vi "Set PORT levels.vi"(8 "error in (no error)":errorcluster, 9 "v (0.000000)":dbl, 10 "i (0)":T1, 11 "VISA resource name":refnum<visa-resource-name>) -> (0 "error out":errorcluster, 3 "VISA resource name out":refnum<visa-resource-name>)   [LabVIEW 2015, in "SR400.lvlib"]
doc: "PL i { ,v }\nThe PL command sets and reads thePORT1 and\nPORT2 output levels. i=1 or 2 to select PORT1 or\nPORT 2 and is required. If v is included, the\noutput level is set to v Volts where -10.000 <= v\n<= 10.000. The resolution is 0.005 V (5 mV). If v\nis absent, the output level is returned. If the Port\noutput mode is SCAN, the PL command sets and\nreads the starting value of the level. Changing the\nlevel during a scan will cause the level to be set to\nthe new value on the next count period. Note that\nthe scan is not reset. Reading the level during a\nscan always returns the starting value, not the\ncurrent value."
uses:
  SR400.lvlib
  Typedefs/PORT Output.ctl
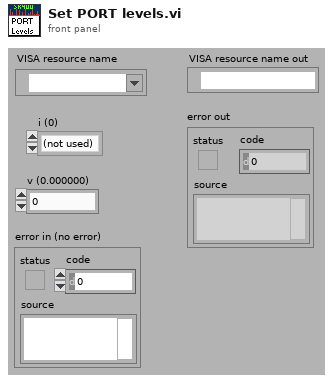
[diagram p1: front panel]
types:
  T1 = typedef "SR400.lvlib/PORT Output.ctl" = enum16{"(not used)", "PORT 1", "PORT 2"}
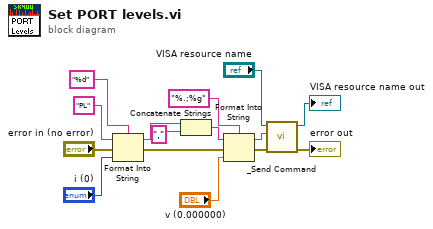
[diagram p0: block diagram]
diagram:
  n1 = Format Into String(format string="%d", initial string="PL" ("command"), error in="error in (no error)", "i (0)") -> (resulting string=w12:string, error out=w13:errorcluster)
  n2 = Concatenate Strings(w12, "," ("command")) -> (w7:string)
  n3 = Format Into String(format string="%.;%g", initial string=w7, error in=w13, "v (0.000000)") -> (resulting string=w4:string, error out=w3:errorcluster)
  n4 = call "_Send Command.vi"("error in (no error)"=w3, "Command"=w4, "VISA resource name"="VISA resource name") -> ("error out"=→"error out":errorcluster, "VISA resource name out"=→"VISA resource name out":refnum<visa-resource-name>)  [unwired: 1 in, 6 out]
